vi "Example 8 - Fault Injection.vi"() -> ()   [LabVIEW 2021]
uses:
  Omni-Bus/Omni_Bus.lvclass
  Omni-Bus/Support/Broad Types.ctl
  Local Bus/Local Bus.lvclass
  C:/Users/Tim/Documents/GitHub/Omni-Bus/Source/Omni-Bus/Bus Access/Bus_Access.lvclass
  <vilib>/Utility/Data Type/Type Definitions/Data Type.ctl
  Aggregator Bus/Aggregator Bus.lvclass
  <vilib>/TSA/Abstract Data Classes/Abs_Types/Type/Abs_Type.lvclass/Abs_Type.ctl
  Omni-Bus/Omni_Bus.lvclass/Omni_Bus.ctl
  Omni-Bus/Support/Write/Write DBL.vi
  Omni-Bus/Support/Read/Read DBL.vi
  Omni-Bus/Support/FindVar.vi
  <vilib>/Utility/error.llb/Clear Errors.vi
  Omni-Bus/Properties/Read Var Map.vi
  <vilib>/TSA/Abstract Data Classes/Abs_Types/Type/Properties/Read Tag.vi
  <vilib>/TSA/Abstract Data Classes/Constants/Support/DBL/Const_DBL.lvclass
  C:/Program Files (x86)/National Instruments/LabVIEW 2021/vi.lib/TSA/Abstract Data Classes/Abs_Types/Type/Abs_Type.lvclass
  <vilib>/TSA/Abstract Data Classes/Abs_Types/Double Float/Abs_Double Float.lvclass
  <vilib>/TSA/Abstract Data Classes/Abs_Types/Value/Abs_Value.lvclass
  <vilib>/TSA/Abstract Data Classes/Constants/Support/DBL/DBL.vi
  Omni-Bus/Support/Check For Read Only Error.vi
  Omni-Bus/Support/Incorrect Tag String Error.vi
  <vilib>/TSA/Abstract Data Classes/Abs_Types/Type/Abs_Type.lvclass
  <vilib>/Utility/Data Type/NI_Data Type.lvlib
  Fault-Injection Bus/Fault-Injection Bus.lvclass
  Fault-Injection Bus/Support/Omni-Bus/Omni-Bus Inject DBL.vi
  C:/Program Files (x86)/National Instruments/LabVIEW 2021/vi.lib/TSA/Abstract Data Classes/Abs_Types/Double Float/Abs_Double Float.lvclass
  C:/Program Files (x86)/National Instruments/LabVIEW 2021/vi.lib/TSA/Abstract Data Classes/Abs_Types/Floating Point/Abs_Floating Point.lvclass
  C:/Program Files (x86)/National Instruments/LabVIEW 2021/vi.lib/TSA/Abstract Data Classes/Abs_Types/Numeric/Abs_Numeric.lvclass
  C:/Program Files (x86)/National Instruments/LabVIEW 2021/vi.lib/TSA/Abstract Data Classes/Abs_Types/Value/Abs_Value.lvclass
  C:/Program Files (x86)/National Instruments/LabVIEW 2021/vi.lib/TSA/Abstract Data Classes/Constants/Support/DBL/Const_DBL.lvclass
  C:/Program Files (x86)/National Instruments/LabVIEW 2021/vi.lib/TSA/Abstract Data Classes/Constants/Support/Interface/Const_Intf.lvclass
  C:/Users/Tim/Documents/GitHub/Omni-Bus/Source/Local Bus/Local Bus.lvclass
  C:/Users/Tim/Documents/GitHub/Omni-Bus/Source/Aggregator Bus/Aggregator Bus.lvclass
  C:/Users/Tim/Documents/GitHub/Omni-Bus/Source/Fault-Injection Bus/Fault-Injection Bus.lvclass
panel:
  in  "Enable 3":bool
  in  "Enable 2":bool
  in  "Enable 1":bool
  out "Fault Injection DBL error 3":errorcluster
  out "Fault Injection DBL error 2":errorcluster
  out "Fault Injection DBL error 1":errorcluster
  in  "Injected Val 3":dbl
  in  "Injected Val 2":dbl
  in  "Injected Val 1":dbl
  in  "Fault Injection DBL Tag 3":string(combo)
  in  "Fault Injection DBL Tag 2":string(combo)
  in  "Fault Injection DBL Tag 1":string(combo)
  in  "Fault Injection Arm":bool
  out "Numeric 4":dbl
  out "Numeric 3":dbl
  in  "Numeric 2":dbl
  in  "Numeric":dbl
  in  "Write DBL Tag":string(combo)
  out "Write DBL error":errorcluster
  in  "Write DBL Tag":string(combo)
  out "Write DBL error":errorcluster
  out "Read DBL Error":errorcluster
  out "Read DBL error":errorcluster
  in  "Read DBL Tag":string(combo)
  in  "Read DBL Tag":string(combo)
  out "Read DBL error":errorcluster
  out "Write DBL error":errorcluster
  in  "Double":dbl
  in  "Write DBL Tag":string(combo)
  in  "stop":bool
  out "Double":dbl format="%.2f"
  in  "Read DBL Tag":string(combo)
  out "error out":errorcluster
  out "All Tags":string[](array[string])
  # "Arm is a Global Enable for\nFault Injection"
  # "Fault Injection Bus\nTakes all of the objects\ncreated by the other buses\nand wraps them in the\nFault Injection Objects, to add\nthe Fault Injection Features."
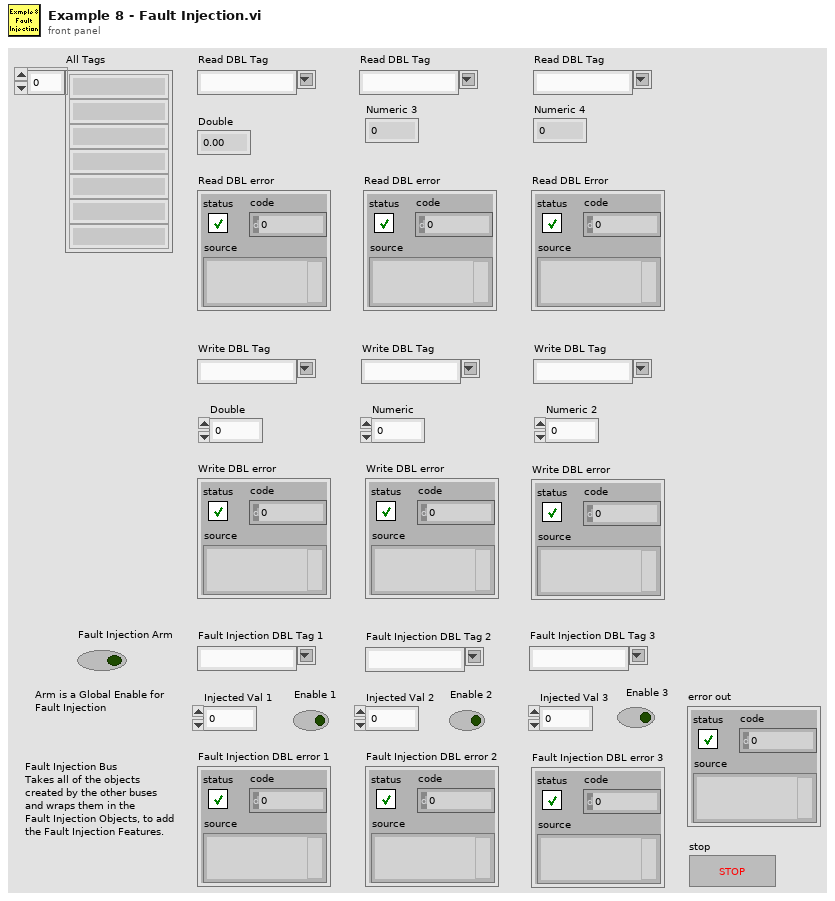
[diagram p1: front panel]
types:
  T1 = typedef "NI_Data Type.lvlib/Data Type.ctl" = enum8{"Invalid Type", "Void", "I8", "I16", "I32", "I64", "U8", "U16", "U32", "U64", "Single Float", "Double Float", "Extended Float", "Single Complex", "Double Complex", "Extended Complex", "Enum U8", "Enum U16", "Enum U32", "Enum U64", "Single Float With Unit", "Double Float With Unit", "Extended Float With Unit", "Single Complex with Unit", "Double Complex with Unit", "Extended Complex with Unit", "Boolean", "String", "Path", "Picture", "Tag", "Array", "Cluster", "Variant", "LV Variant", "Waveform", "Timestamp", "Digital Waveform", "Digital Data", "ExpressData", "Refnum", "External Data", "VI", "Poly VI", "LabVIEW Class Instance", "Fixed Point", "Set Collection", "Map Collection"}
  T2 = typedef "Omni_Bus.lvclass/Broad Types.ctl" = enum16{"All Tags", "NI Specific Type", "Boolean", "String", "Numeric", "Float", "Integer", "Collection", "All Value Types", "Non Value Types"}
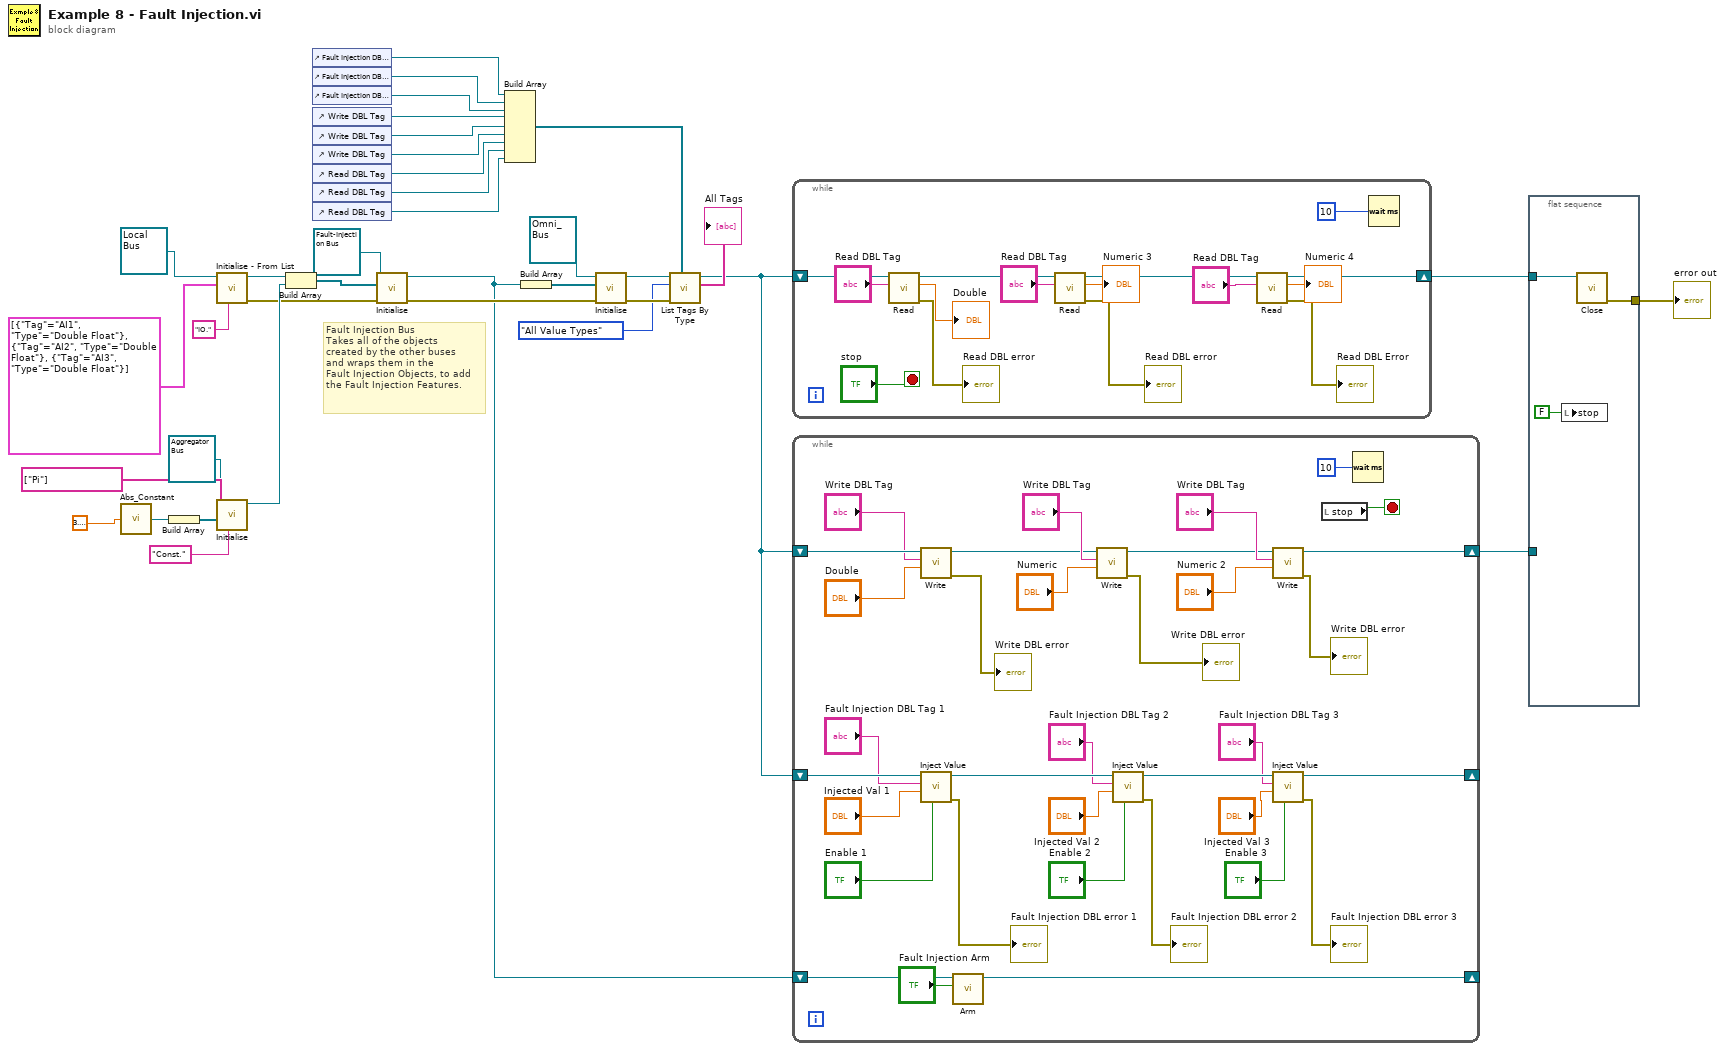
[diagram p0: block diagram]
diagram:
  # "Fault Injection Bus\nTakes all of the objects\ncreated by the other buses\nand wraps them in the\nFault Injection Objects, to add\nthe Fault Injection Features."
  n1 = call-poly <vilib>:"Abs_Constant.vi"("Value"=3.141592653589793) -> ("Constant"=w23:refnum<class "Const_DBL.lvclass">)  [unwired: 4 in]
  n2 = Build Array(w23) -> (w24:refnum<class "Const_DBL.lvclass">[])
  n3 = call "Initialise - From List.vi"("Tag Root"="IO.", "Tag List"=cluster{"Tag":string, "Type":T1}[] [{"Tag"="AI1", "Type"=enum."Double Float"}, {"Tag"="AI2", "Type"=enum."Double Float"}, {"Tag"="AI3", "Type"=enum."Double Float"}], "Local Bus in"=refnum<class "Local Bus.lvclass"> refnum ("Local Bus.lvclass")) -> ("error out"=w8:errorcluster, "Local Bus out"=w28:refnum<class "Local Bus.lvclass">)  [unwired: 7 in]
  n4 = call "Initialise.vi"("Tag Root"="Const.", "Values"=w24, "Tags"=string[] ["Pi"], "Aggregator Bus in"=refnum<class "Aggregator Bus.lvclass"> refnum) -> ("Aggregator Bus out"=w25:refnum<class "Aggregator Bus.lvclass">)  [unwired: 6 in, 1 out]
  n5 = Build Array(w28, w25) -> (w9:refnum<class "Bus_Access.lvclass">[])
  n6 = control-ref of="Fault Injection DBL Tag 1"() -> (w1:refnum<vi>)
  n7 = control-ref of="Fault Injection DBL Tag 2"() -> (w2:refnum<vi>)
  n8 = control-ref of="Fault Injection DBL Tag 3"() -> (w3:refnum<vi>)
  n9 = control-ref of="Write DBL Tag"() -> (w18:refnum<vi>)
  n10 = control-ref of="Write DBL Tag"() -> (w17:refnum<vi>)
  n11 = control-ref of="Write DBL Tag"() -> (w16:refnum<vi>)
  n12 = control-ref of="Read DBL Tag"() -> (w15:refnum<vi>)
  n13 = control-ref of="Read DBL Tag"() -> (w14:refnum<vi>)
  n14 = control-ref of="Read DBL Tag"() -> (w13:refnum<vi>)
  n15 = call "Initialise.vi"("error in (no error)"=w8, "Buses"=w9, "Fault-Injection Bus in"=refnum<class "Fault-Injection Bus.lvclass"> refnum) -> ("error out"=w7:errorcluster, "Fault-Injection Bus out"=w4:refnum<class "Fault-Injection Bus.lvclass">)  [unwired: 7 in]
  n16 = Build Array(w1, w2, w3, w18, w17, w16, w15, w14, w13) -> (w12:refnum<vi>[])
  n17 = Build Array(w4) -> (w20:refnum<class "Fault-Injection Bus.lvclass">[])
  n18 = call-dynamic "Initialise.vi"("error in (no error)"=w7, "Bus Access"=w20, "Var Bus in"=refnum<class "Omni_Bus.lvclass"> refnum) -> ("error out"=w34:errorcluster, "Var Bus out"=w35:refnum<class "Omni_Bus.lvclass">)  [unwired: 7 in]
  n19 = call "List Tags By Type.vi"("Combo Boxes"=w12, "error in (no error)"=w34, "Broad Types"=Broad_Types."All Value Types", "Var Bus in"=w35) -> ("Tags"=→"All Tags":string[], "Var Bus out"=w5:refnum<class "Omni_Bus.lvclass">)  [unwired: 4 in, 2 out]
  n20 = while {
    shift-right: [w41] -> w30
    shift-left: w5 -> [w51]
    stop <- "stop" stop-if-true
    n21 = call-poly "Read.vi"("Tag"="Read DBL Tag", "Var Bus in"=w51) -> ("error out"=→"Read DBL error":errorcluster, "Numeric"=→"Double":dbl, "Var Bus out"=w44:refnum<class "Omni_Bus.lvclass">)  [unwired: 7 in]
    n22 = call-poly "Read.vi"("Tag"="Read DBL Tag", "Var Bus in"=w44) -> ("error out"=→"Read DBL error":errorcluster, "Numeric"=→"Numeric 3":dbl, "Var Bus out"=w42:refnum<class "Omni_Bus.lvclass">)  [unwired: 7 in]
    n23 = call-poly "Read.vi"("Tag"="Read DBL Tag", "Var Bus in"=w42) -> ("error out"=→"Read DBL Error":errorcluster, "Numeric"=→"Numeric 4":dbl, "Var Bus out"=w41:refnum<class "Omni_Bus.lvclass">)  [unwired: 7 in]
    n24 = Wait (ms)(milliseconds to wait=u32 10) -> ()  [unwired: 1 out]
  }
  n25 = while {
    shift-right: [w73] -> w29
    shift-left: w5 -> [w85]
    shift-right: [w64] -> _
    shift-left: w5 -> [w70]
    shift-right: [w68] -> _
    shift-left: w4 -> [w69]
    stop <- w82 stop-if-true
    n26 = call-poly "Write.vi"("Numeric"="Double", "Tag"="Write DBL Tag", "Omni_Bus in"=w85) -> ("error out"=→"Write DBL error":errorcluster, "Omni_Bus out"=w77:refnum<class "Omni_Bus.lvclass">)  [unwired: 7 in]
    n27 = call-poly "Inject Value.vi"("Enable"="Enable 1", "Injected Value"="Injected Val 1", "Tag"="Fault Injection DBL Tag 1", "Omni_Bus in"=w70) -> ("error out"=→"Fault Injection DBL error 1":errorcluster, "Omni_Bus out"=w66:refnum<class "Omni_Bus.lvclass">)  [unwired: 6 in]
    n28 = call "Arm.vi"("Arm"="Fault Injection Arm", "Fault-Injection Bus in"=w69) -> ("Fault-Injection Bus out"=w68:refnum<class "Fault-Injection Bus.lvclass">)  [unwired: 8 in, 1 out]
    n29 = call-poly "Write.vi"("Numeric"="Numeric", "Tag"="Write DBL Tag", "Omni_Bus in"=w77) -> ("error out"=→"Write DBL error":errorcluster, "Omni_Bus out"=w74:refnum<class "Omni_Bus.lvclass">)  [unwired: 7 in]
    n30 = call-poly "Inject Value.vi"("Enable"="Enable 2", "Injected Value"="Injected Val 2", "Tag"="Fault Injection DBL Tag 2", "Omni_Bus in"=w66) -> ("error out"=→"Fault Injection DBL error 2":errorcluster, "Omni_Bus out"=w65:refnum<class "Omni_Bus.lvclass">)  [unwired: 6 in]
    n31 = call-poly "Write.vi"("Numeric"="Numeric 2", "Tag"="Write DBL Tag", "Omni_Bus in"=w74) -> ("error out"=→"Write DBL error":errorcluster, "Omni_Bus out"=w73:refnum<class "Omni_Bus.lvclass">)  [unwired: 7 in]
    n32 = call-poly "Inject Value.vi"("Enable"="Enable 3", "Injected Value"="Injected Val 3", "Tag"="Fault Injection DBL Tag 3", "Omni_Bus in"=w65) -> ("error out"=→"Fault Injection DBL error 3":errorcluster, "Omni_Bus out"=w64:refnum<class "Omni_Bus.lvclass">)  [unwired: 6 in]
    n33 = local read "stop"() -> (w82:bool)
    n34 = Wait (ms)(milliseconds to wait=u32 10) -> ()  [unwired: 1 out]
  }
  n35 = flat-sequence {
    tunnel: [w88] -> w31
    tunnel: w30 -> [w87]
    tunnel: w29 -> [_]
    frame #0 {
      n36 = local write "stop"(FALSE ("stop")) -> ()
      n37 = call-dynamic "Close.vi"("Data in"=w87) -> ("error out"=w88:errorcluster)  [unwired: 9 in, 1 out]
    }
  }
  "error out" <- w31
